vi "ImagingSubVI.vi"(1 "Check timings (bool 3)":bool, 2 "Set image (bool 2)":bool) -> (0 "Initialize (bool 1)":bool)   [LabVIEW 2019]
uses:
  <vilib>/Utility/file.llb/Write Delimited Spreadsheet (I64).vi
  Program Files (x86)/National Instruments/LabVIEW 2019/ATMCD32D.dll
panel:
  in  "Tab Control":T1(tab)
  out "Expected position on spectrometer (pixels):":dbl
  in  "Harmonic":dbl min=10.0 max=40.0
  out "l (nm)":dbl
  out "E (J)":dbl
  out "E (eV)":dbl
  out "Nearest Harmonic of 800nm":dbl
  out "Cursor Position (pixels)":dbl
  out "Distance to nearest harmonic of 800nm (pixels)":dbl
  in  "Grating:":u16(ring) items=["Shimadzu 30-006  "]
  in  "Laser:":u16(ring) items=["800nm  "]
  out "Get Acquired Data":u32
  out "Start Acquisition":u32
  in  "Detector X Pixels":i32
  in  "Get Detector":u32
  in  "Detector Y Pixels":i32
  out "Intensity Graph":i32[][](graph)
  out "Vertical Binned Waveform Graph":i32[](graph)
  out "Get Status":u32
  in  "Stop":bool
  in  "?":bool
  out "Camera Status:":bool
  out "Last Image Saved:":string
  out "Wavelength Graph":cluster{"No prefix":dbl, i32}[](graph)
  out "Energy Graph (eV)":cluster{"eV":dbl, i32}[](graph)
  out "Harmonics Graph":cluster{"No prefix":dbl, i32}[](graph)
  out "Status":u32
  # "Status"
  # "Return values"
  # "USB iStarIMAG32at.VI"
  # "Acquisition Mode: Single Scan\nReadout Mode: Full Resolution Image"
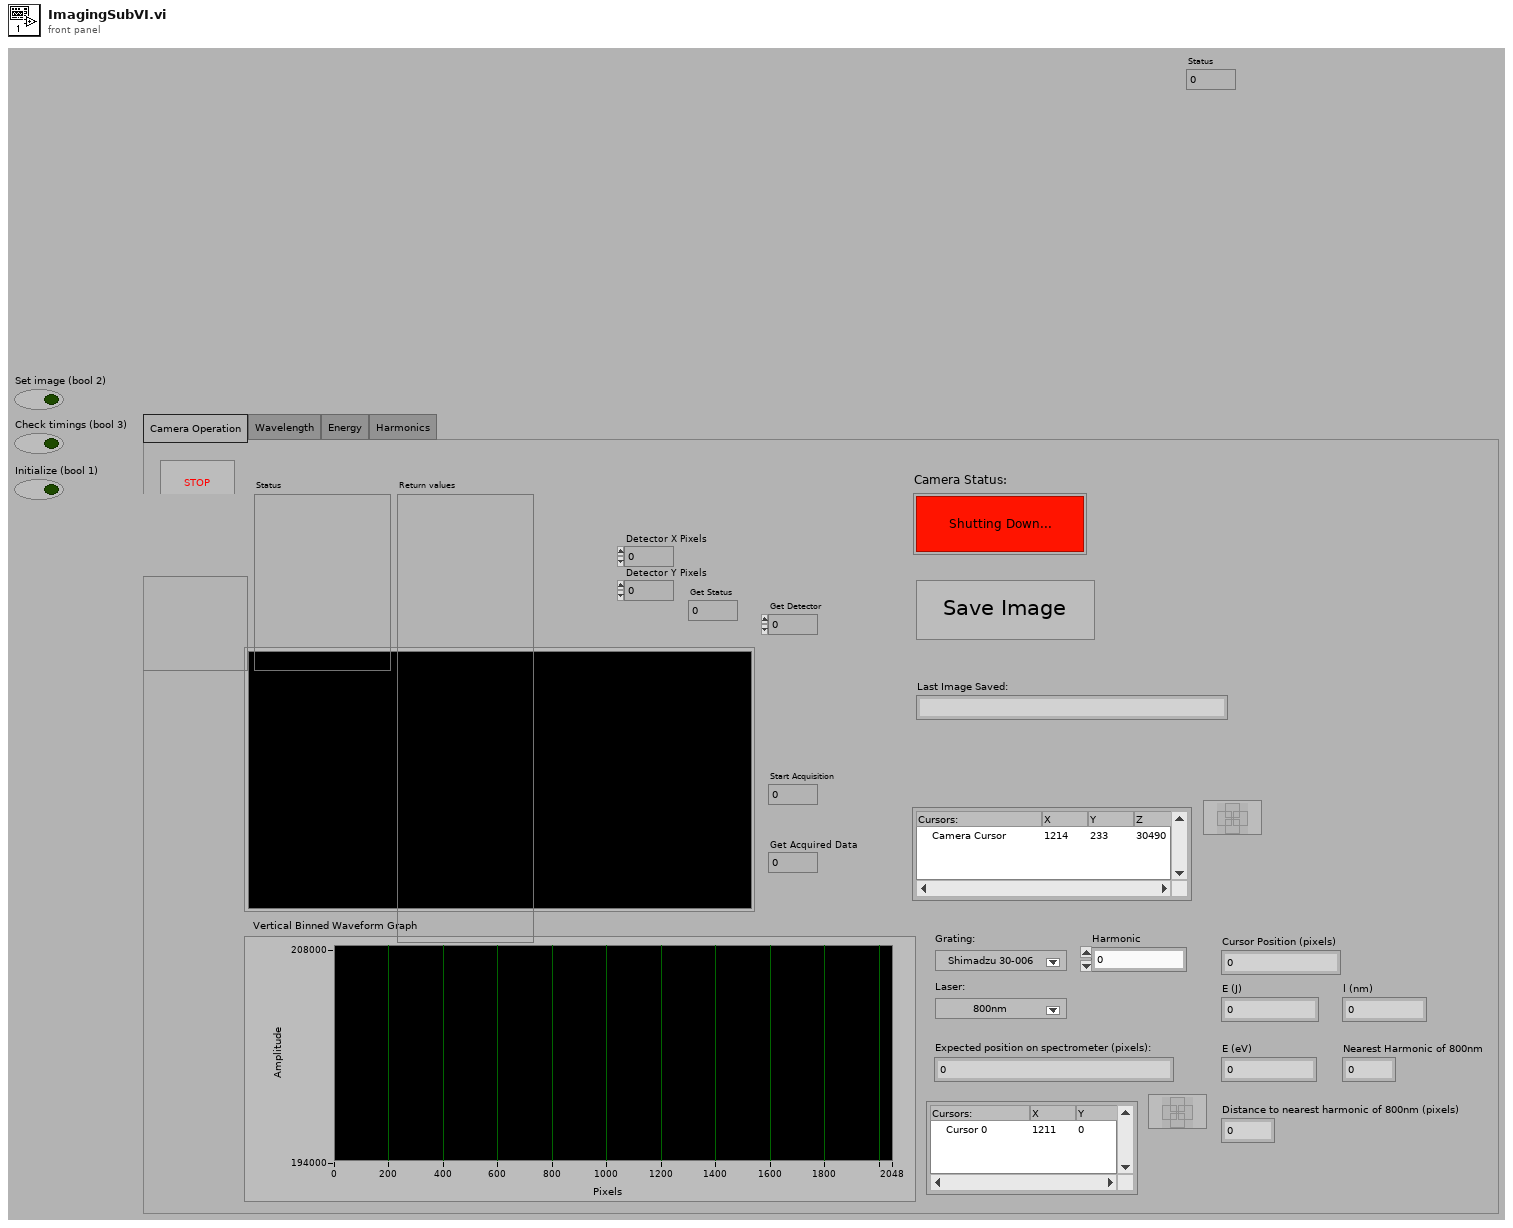
[diagram p1: front panel]
types:
  T1 = enum32{"Camera Operation", "Wavelength", "Energy", "Harmonics"}
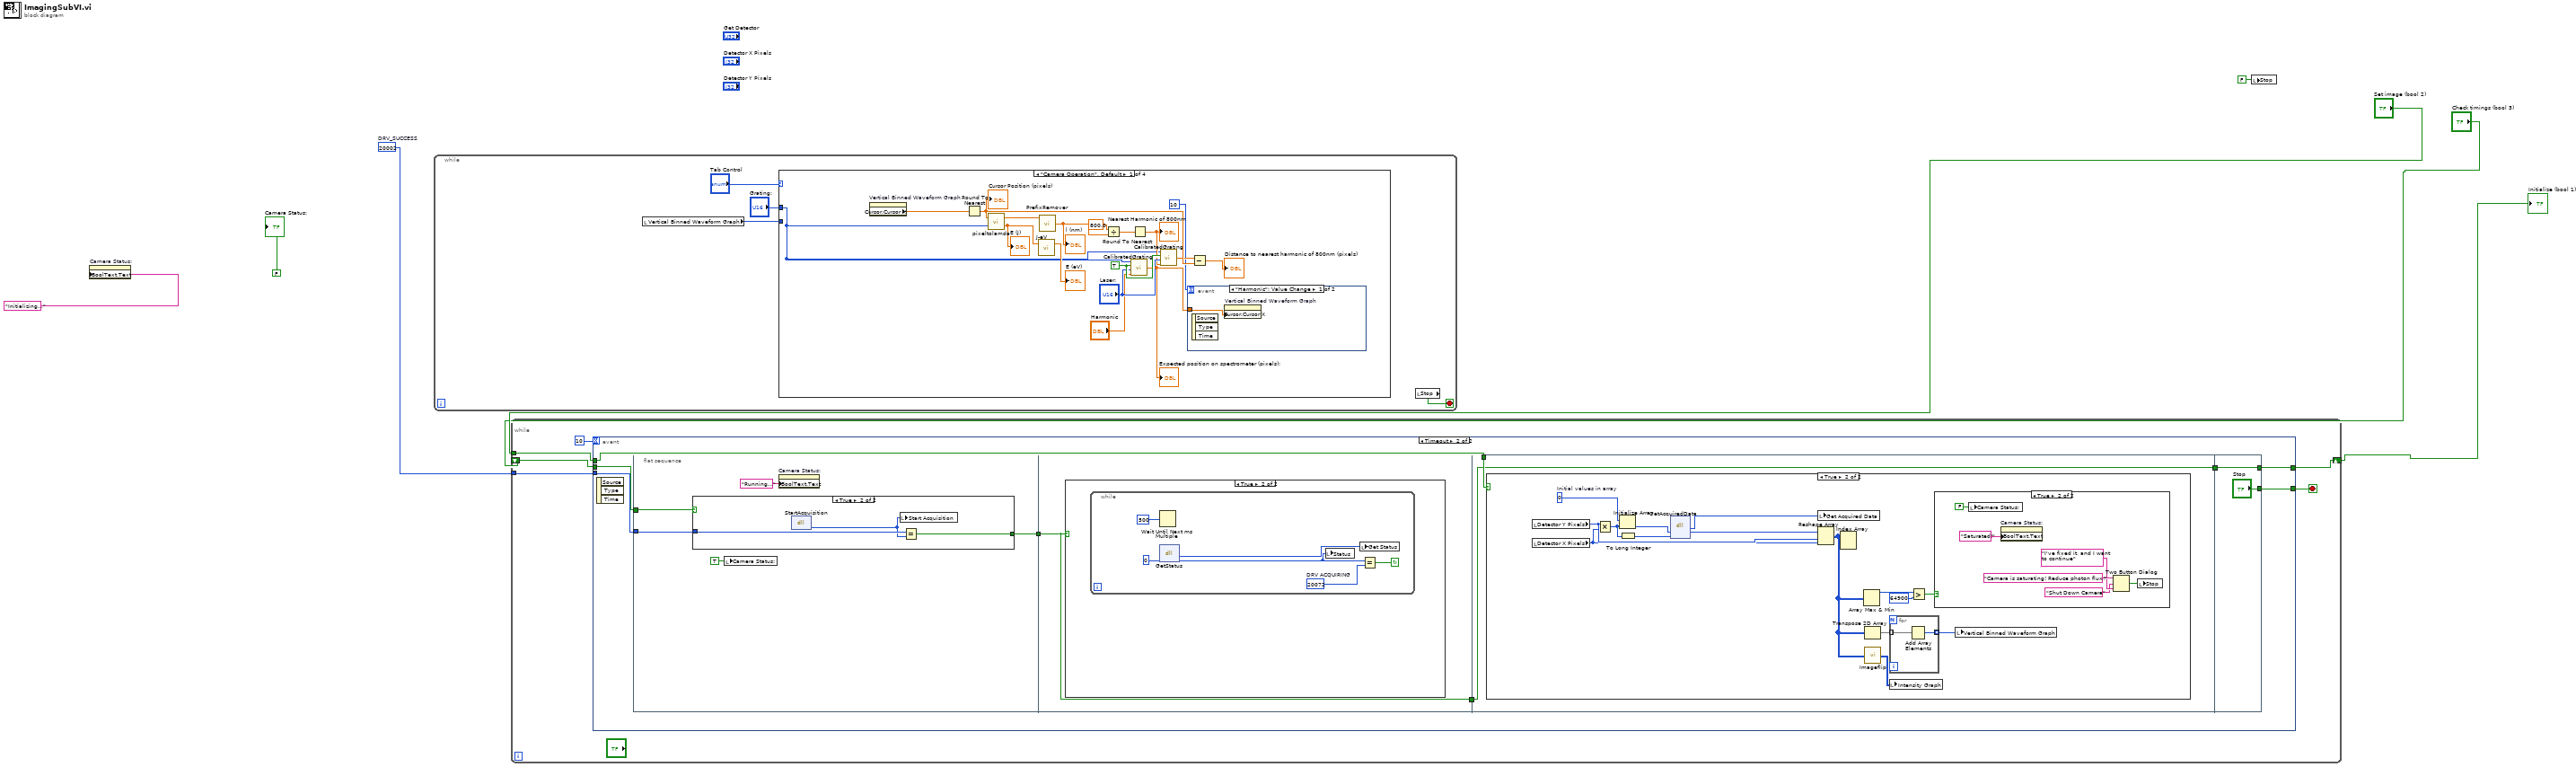
[diagram p0: block diagram]
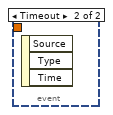
[diagram p2: hidden frame]
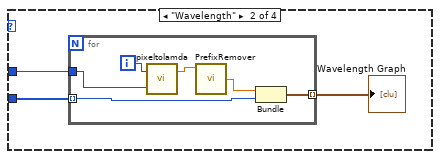
[diagram p3: hidden frame]
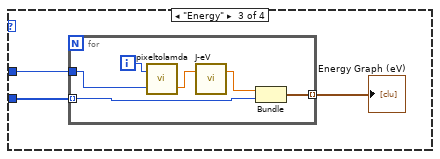
[diagram p4: hidden frame]
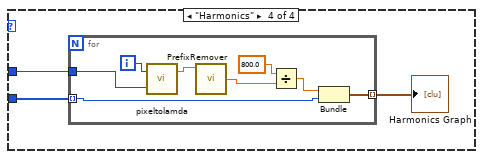
[diagram p5: hidden frame]
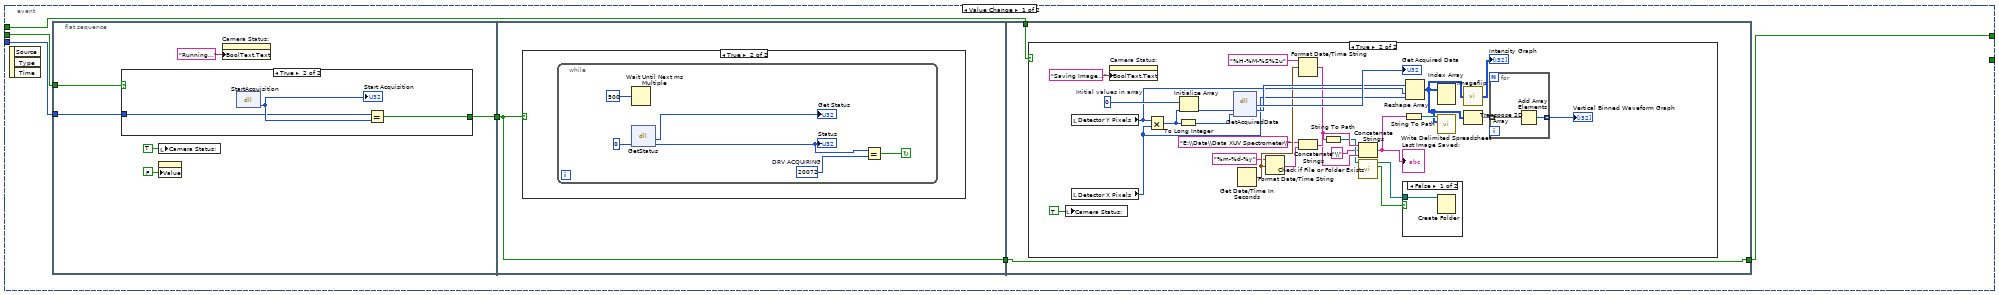
[diagram p6: hidden frame]
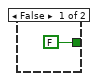
[diagram p7: hidden frame]
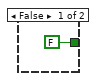
[diagram p11: hidden frame]
diagram:
  w7 = 20002  # DRV_SUCCESS
  n1 = property on="Camera Status:" class="Bool (strict)"("BoolText.Text"="Initializing..." ("String")) -> ()  [unwired: 2 in, 2 out]
  n2 = while {
    stop <- w8 stop-if-true
    n3 = local read "Vertical Binned Waveform Graph"() -> (w10:i32[])
    n4 = case shown="\"Camera Operation\", Default" "Tab Control" {
      tunnel: w10 -> [_ w32 w41 w50]
      tunnel: "Grating:" -> [w12 w31 w40 w49]
      frame "Camera Operation", Default {
        w28 = TRUE
        n5 = property on="Vertical Binned Waveform Graph" class="WFGraph (strict)"() -> ("Cursor.Cursor X"=w25:dbl)  [unwired: 2 in, 2 out]
        n6 = Round To Nearest(number=w25) -> (nearest integer value=w18:dbl)
        "Cursor Position (pixels)" <- w18
        n7 = call "pixeltolamda.vi"("Grating:"=w12, "Pixel Postion"=w18) -> ("E (J)"=w20:dbl, "lamda (m)"=w26:dbl)
        "E (J)" <- w20
        n8 = call "J-eV.vi"("J"=w20) -> ("eV"=→"E (eV)":dbl)  [unwired: 1 in, 1 out]
        n9 = call "PrefixRemover.vi"("Nano"=w26) -> ("No prefix"=w21:dbl)  [unwired: 3 in]
        "l (nm)" <- w21
        n10 = Divide(x=800.0, y=w21) -> (x/y=w23:dbl)
        n11 = call "CalibratedGrating.vi"("Harmonic"="Harmonic", "Laser:"="Laser:", "Subvi?"=w28, "Grating:"=w12) -> ("Position on spectrometer (pixels):"=w14:dbl)
        "Expected position on spectrometer (pixels):" <- w14
        n12 = Round To Nearest(number=w23) -> (nearest integer value=w17:dbl)
        "Nearest Harmonic of 800nm" <- w17
        n13 = call "CalibratedGrating.vi"("Harmonic"=w17, "Laser:"="Laser:", "Subvi?"=w28, "Grating:"=w12) -> ("Position on spectrometer (pixels):"=w16:dbl)
        n14 = event shown="[0] \"Harmonic\": Value Change" {
          selector: _ -> [_ _]
          dyn-events: _ -> [_ _]
          timeout: 10 -> [_ _]
          tunnel: w14 -> [w29 _]
          event "Harmonic": Value Change {
            n15 = event-data() -> ()  [unwired: 1 in, 3 out]
            n16 = property on="Vertical Binned Waveform Graph" class="WFGraph (strict)"("Cursor.Cursor X"=w29) -> ()  [unwired: 2 in, 2 out]
          }
          event Timeout {
            n17 = event-data() -> ()  [unwired: 1 in, 3 out]
          }
        }
        n18 = Subtract(x=w16, y=w18) -> (x-y=→"Distance to nearest harmonic of 800nm (pixels)":dbl)
      }
      frame "Wavelength" {
        n19 = for {
          tunnel: w32 -> [w34] mode=indexing
          tunnel: w31 -> [w36]
          tunnel: [w33] -> w30 mode=indexing
          i -> [w35]
          n20 = call "pixeltolamda.vi"("Grating:"=w36, "Pixel Postion"=w35) -> ("lamda (m)"=w37:dbl)  [unwired: 1 out]
          n21 = call "PrefixRemover.vi"("Nano"=w37) -> ("No prefix"=w38:dbl)  [unwired: 3 in]
          n22 = Bundle("No prefix"=w38, w34) -> (w33:cluster{"No prefix":dbl, i32})  [unwired: 1 in]
        }
        "Wavelength Graph" <- w30
      }
      frame "Energy" {
        n23 = for {
          tunnel: w41 -> [w43] mode=indexing
          tunnel: w40 -> [w46]
          tunnel: [w42] -> w39 mode=indexing
          i -> [w47]
          n24 = call "pixeltolamda.vi"("Grating:"=w46, "Pixel Postion"=w47) -> ("E (J)"=w45:dbl)  [unwired: 1 out]
          n25 = call "J-eV.vi"("J"=w45) -> ("eV"=w44:dbl)  [unwired: 1 in, 1 out]
          n26 = Bundle("eV"=w44, w43) -> (w42:cluster{"eV":dbl, i32})  [unwired: 1 in]
        }
        "Energy Graph (eV)" <- w39
      }
      frame "Harmonics" {
        n27 = for {
          tunnel: w50 -> [w55] mode=indexing
          tunnel: w49 -> [w57]
          tunnel: [w54] -> w48 mode=indexing
          i -> [w56]
          n28 = call "pixeltolamda.vi"("Grating:"=w57, "Pixel Postion"=w56) -> ("lamda (m)"=w58:dbl)  [unwired: 1 out]
          n29 = call "PrefixRemover.vi"("Nano"=w58) -> ("No prefix"=w52:dbl)  [unwired: 3 in]
          n30 = Divide(x=800.0, y=w52) -> (x/y=w51:dbl)
          n31 = Bundle(w51, w55) -> (w54:cluster{dbl, i32})  [unwired: 1 in]
        }
        "Harmonics Graph" <- w48
      }
    }
    n32 = local read "Stop"() -> (w8:bool)
  }
  n33 = while {
    tunnel: w7 -> [w63]
    tunnel: "Set image (bool 2)" -> [w61]
    shift-right: [w62] -> w1
    shift-left: "Check timings (bool 3)" -> [w64]
    stop <- w59 stop-if-true
    n34 = event shown="[1] Timeout" {
      selector: _ -> [_ _]
      dyn-events: _ -> [_ _]
      timeout: 10 -> [_ _]
      tunnel: w64 -> [w68 w125]
      tunnel: w63 -> [w67 w124]
      tunnel: [w66 w123] -> w62
      tunnel: w61 -> [w65 w122]
      tunnel: [_ w121] -> w59
      event Value Change {
        n35 = event-data() -> ()  [unwired: 1 in, 3 out]
        n36 = flat-sequence {
          tunnel: w68 -> [w76]
          tunnel: w67 -> [w75]
          tunnel: [w74] -> w70
          tunnel: w70 -> [w81]
          tunnel: [w81] -> w69
          tunnel: [w89] -> w66
          tunnel: w69 -> [w89]
          tunnel: w65 -> [w88]
          frame #0 {
            n37 = case shown="True" w76 {
              tunnel: [FALSE w79] -> w74
              tunnel: w75 -> [_ w78]
              frame False {
              }
              frame True {
                n38 = dll-call lib="C:/Program Files (x86)/National Instruments/LabVIEW 2019/atmcd32d.dll" fn="StartAcquisition" label="Call Library Function start acquisition"() -> (w80:u32)  [unwired: 3 in, 2 out]
                "Start Acquisition" <- w80
                n39 = Equal?(x=w78, y=w80) -> (x = y?=w79:bool)
              }
            }
            n40 = local write "Camera Status:"(TRUE ("Camera Status:")) -> ()
            n41 = property class="Bool (strict)"("Value"=FALSE ("Take image")) -> ()  [unwired: 2 in, 2 out]
            n42 = property on="Camera Status:" class="Bool (strict)"("BoolText.Text"="Running..." ("Boolean Text.Text")) -> ()  [unwired: 2 in, 2 out]
          }
          frame #1 {
            n43 = case shown="True" w81 {
              frame False {
              }
              frame True {
                n44 = while {
                  stop <- w85 continue-if-true
                  w84 = u16 20072  # DRV ACQUIRING
                  n45 = Wait Until Next ms Multiple(millisecond multiple=u32 500) -> ()  [unwired: 1 out]
                  n46 = dll-call lib="C:/Program Files (x86)/National Instruments/LabVIEW 2019/atmcd32d.dll" fn="GetStatus" label="Call Library Function GetAcquisitionStatus"(u16 0) -> (→"Get Status":u32, w83:u32)  [unwired: 3 in, 2 out]
                  "Status" <- w83
                  n47 = Equal?(x=w83, y=w84) -> (x = y?=w85:bool)
                }
              }
            }
          }
          frame #2 {
            n48 = case shown="True" w88 {
              frame False {
              }
              frame True {
                w116 = 0  # Initial values in array
                n49 = local write "Camera Status:"(TRUE ("Camera Status:")) -> ()
                n50 = local read "Detector Y Pixels"() -> (w110:i32)
                n51 = local read "Detector X Pixels"() -> (w109:i32)
                n52 = property on="Camera Status:" class="Bool (strict)"("BoolText.Text"="Saving Image..." ("Boolean Text.Text")) -> ()  [unwired: 2 in, 2 out]
                n53 = Multiply(x=w110, y=w109) -> (x*y=w112:i32)
                n54 = To Long Integer(number=w112) -> (32bit integer=w113:i32)
                n55 = Initialize Array "Initialize Array"(w116, w112) -> (w114:i32[])
                n56 = dll-call lib="C:/Program Files (x86)/National Instruments/LabVIEW 2019/atmcd32d.dll" fn="GetAcquiredData" label="Call Library Function Get Acquired data"(w114, w113) -> (→"Get Acquired Data":u32, w111:i32[])  [unwired: 4 in, 2 out]
                n57 = Get Date/Time In Seconds() -> (seconds since 1Jan1904=w106:timestamp)
                n58 = Format Date/Time String(time format string (%c)="%m-%d-%y", seconds (now)=w106) -> (date/time string=w104:string)  [unwired: 1 in]
                n59 = Format Date/Time String(time format string (%c)="%H-%M-%S%2u", seconds (now)=w106) -> (date/time string=w105:string)  [unwired: 1 in]
                n60 = Concatenate Strings("E:\\Data\\Data XUV Spectrometer\\" ("string"), w104) -> (w107:string)
                n61 = String To Path(string=w107) -> (path=w103:path)
                n62 = Concatenate Strings(w107, "\\" ("string"), w105) -> (w108:string)
                "Last Image Saved:" <- w108
                n63 = call <vilib>:"Check if File or Folder Exists.vi"("path"=w103) -> ("file or folder exists?"=w101:bool, "dup path"=w102:path)  [unwired: 8 in, 1 out]
                n64 = case shown="False" w101 {
                  tunnel: w102 -> [w119 _]
                  frame False {
                    n65 = Create Folder(path (use dialog)=w119) -> ()  [unwired: 2 in, 3 out]
                  }
                  frame True {
                  }
                }
                n66 = String To Path(string=w108) -> (path=w96:path)
                n67 = Reshape Array(w111, w110, w109) -> (w91:i32[][])
                n68 = Index Array(array=w91) -> ()  [unwired: 2 in, 1 out]
                n69 = call-poly <vilib>:"Write Delimited Spreadsheet.vi"("file path (dialog if empty)"=w96, "2D data"=w91) -> ()  [unwired: 12 in, 2 out]
                n70 = call "Imageflip.vi"("2D array"=w91) -> ("transposed array"=→"Intensity Graph":i32[][])
                n71 = Transpose 2D Array(2D array=w91) -> (transposed array=w95:i32[][])
                n72 = for {
                  tunnel: w95 -> [w118] mode=indexing
                  tunnel: [w117] -> w94 mode=indexing
                  n73 = Add Array Elements(numeric array=w118) -> (sum=w117:i32)
                }
                "Vertical Binned Waveform Graph" <- w94
              }
            }
          }
        }
      }
      event Timeout {
        n74 = event-data() -> ()  [unwired: 1 in, 3 out]
        n75 = flat-sequence {
          tunnel: w125 -> [w132]
          tunnel: w124 -> [w131]
          tunnel: [w130] -> w127
          tunnel: w127 -> [w137]
          tunnel: [w137] -> w126
          tunnel: w126 -> [w144]
          tunnel: w122 -> [w145]
          tunnel: [w144] -> w120
          tunnel: ["Stop"] -> w121
          tunnel: [w170] -> w123
          tunnel: w120 -> [w170]
          frame #0 {
            n76 = case shown="True" w132 {
              tunnel: [FALSE w136] -> w130
              tunnel: w131 -> [_ w135]
              frame False {
              }
              frame True {
                n77 = dll-call lib="C:/Program Files (x86)/National Instruments/LabVIEW 2019/atmcd32d.dll" fn="StartAcquisition" label="Call Library Function start acquisition"() -> (w134:u32)  [unwired: 3 in, 2 out]
                n78 = local write "Start Acquisition"(w134) -> ()
                n79 = Equal?(x=w135, y=w134) -> (x = y?=w136:bool)
              }
            }
            n80 = local write "Camera Status:"(TRUE ("Camera Status:")) -> ()
            n81 = property on="Camera Status:" class="Bool (strict)"("BoolText.Text"="Running..." ("Boolean Text.Text")) -> ()  [unwired: 2 in, 2 out]
          }
          frame #1 {
            n82 = case shown="True" w137 {
              frame False {
              }
              frame True {
                n83 = while {
                  stop <- w141 continue-if-true
                  w140 = u16 20072  # DRV ACQUIRING
                  n84 = Wait Until Next ms Multiple(millisecond multiple=u32 500) -> ()  [unwired: 1 out]
                  n85 = dll-call lib="C:/Program Files (x86)/National Instruments/LabVIEW 2019/atmcd32d.dll" fn="GetStatus" label="Call Library Function GetAcquisitionStatus"(u16 0) -> (w139:u32, w138:u32)  [unwired: 3 in, 2 out]
                  n86 = local write "Status"(w138) -> ()
                  n87 = local write "Get Status"(w139) -> ()
                  n88 = Equal?(x=w138, y=w140) -> (x = y?=w141:bool)
                }
              }
            }
          }
          frame #2 {
            n89 = case shown="True" w145 {
              frame False {
              }
              frame True {
                w160 = 0  # Initial values in array
                n90 = local read "Detector Y Pixels"() -> (w155:i32)
                n91 = local read "Detector X Pixels"() -> (w154:i32)
                n92 = Multiply(x=w155, y=w154) -> (x*y=w157:i32)
                n93 = Initialize Array "Initialize Array"(w160, w157) -> (w159:i32[])
                n94 = To Long Integer(number=w157) -> (32bit integer=w158:i32)
                n95 = dll-call lib="C:/Program Files (x86)/National Instruments/LabVIEW 2019/atmcd32d.dll" fn="GetAcquiredData" label="Call Library Function Get Acquired data"(w159, w158) -> (w152:u32, w156:i32[])  [unwired: 4 in, 2 out]
                n96 = local write "Get Acquired Data"(w152) -> ()
                n97 = Reshape Array(w156, w155, w154) -> (w146:i32[][])
                n98 = Index Array(array=w146) -> ()  [unwired: 2 in, 1 out]
                n99 = Array Max & Min(array=w146) -> (max value=w150:i32)  [unwired: 3 out]
                n100 = Transpose 2D Array(2D array=w146) -> (transposed array=w153:i32[][])
                n101 = call "Imageflip.vi"("2D array"=w146) -> ("transposed array"=w147:i32[][])
                n102 = for {
                  tunnel: w153 -> [w168] mode=indexing
                  tunnel: [w167] -> w151 mode=indexing
                  n103 = Add Array Elements(numeric array=w168) -> (sum=w167:i32)
                }
                n104 = local write "Intensity Graph"(w147) -> ()
                n105 = Greater?(x=w150, y=64900) -> (0:w148:bool)
                n106 = case shown="True" w148 {
                  frame False {
                  }
                  frame True {
                    n107 = local write "Camera Status:"(FALSE ("Camera Status:")) -> ()
                    n108 = property on="Camera Status:" class="Bool (strict)"("BoolText.Text"="Saturated!" ("Boolean Text.Text")) -> ()  [unwired: 2 in, 2 out]
                    n109 = Two Button Dialog(message="Camera is saturating! Reduce photon flux!", 1:"I've fixed it, and I want to continue" ("message"), 2:"Shut Down Camera" ("T button name (\"OK\")")) -> (T button?=w162:bool)
                    n110 = local write "Stop"(w162) -> ()
                  }
                }
                n111 = local write "Vertical Binned Waveform Graph"(w151) -> ()
              }
            }
          }
          frame #3 {
          }
        }
      }
    }
  }
  "Initialize (bool 1)" <- w1
  n112 = local write "Stop"(FALSE ("Stop")) -> ()
  "Camera Status:" <- FALSE ("Camera Status:")
